vi "Launch Set Up.vi"(8 "error in (no error)":errorcluster, 11 "name or relative path":string) -> (0 "error out":errorcluster, 3 "appended path":path)   [LabVIEW 2012]
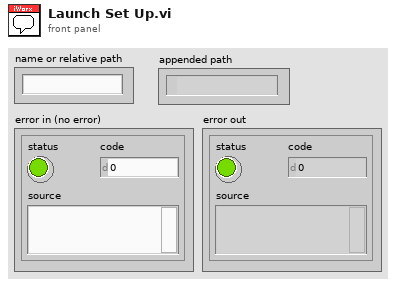
[diagram p1: front panel]
types:
  T1 = enum32{"Invalid", "Standard", "Closed", "Hidden", "Minimized", "Maximized"}
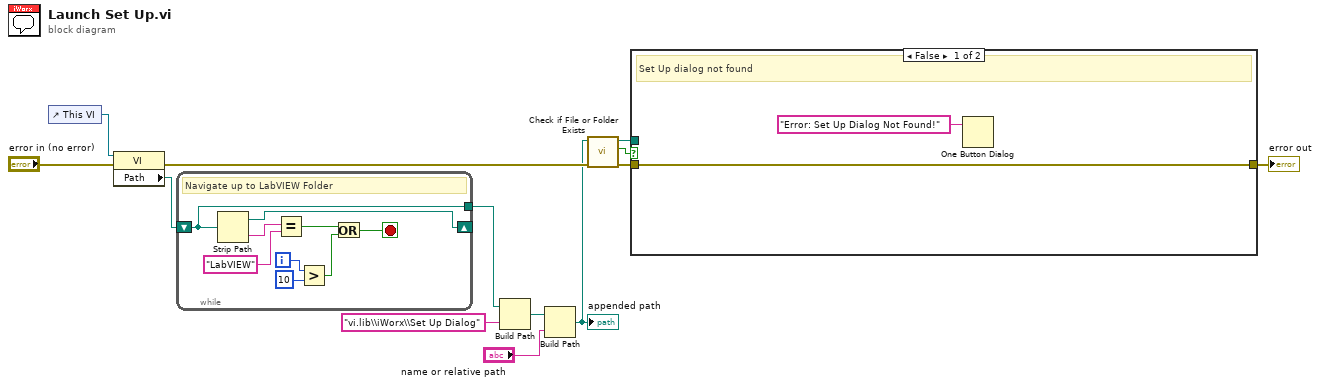
[diagram p0: block diagram]
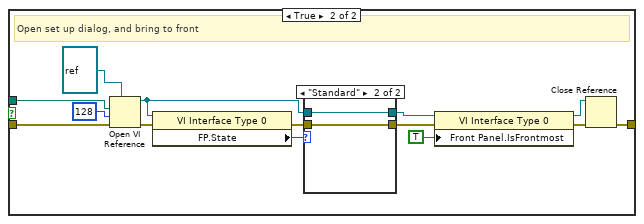
[diagram p2: hidden frame]
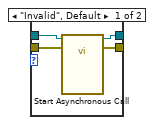
[diagram p3: hidden frame]
diagram:
  n1 = control-ref of="This VI"() -> (w8:refnum<vi>)
  n2 = property class="VI"(reference=w8, error in="error in (no error)") -> (error out=w5:errorcluster, "Path"=w9:path)  [unwired: 1 out]
  n3 = while {
    shift-right: [w22] -> _
    shift-left: w9 -> [w19]
    tunnel: [w19] -> w12
    i -> [w17]
    stop <- w14 stop-if-true
    # "Navigate up to LabVIEW Folder"
    n4 = Strip Path(path=w19) -> (stripped path=w22:path, name=w21:string)
    n5 = Equal?(x=w21, y="LabVIEW" ("name or relative path")) -> (x = y?=w18:bool)
    n6 = Greater?(x=w17, y=10) -> (0:w15:bool)
    n7 = Or(x=w18, y=w15) -> (x .or. y?=w14:bool)
  }
  n8 = Build Path(base path=w12, name or relative path="vi.lib\\iWorx\\Set Up Dialog") -> (appended path=w13:path)
  n9 = Build Path(base path=w13, name or relative path="name or relative path") -> (appended path=w4:path)
  "appended path" <- w4
  n10 = call <vilib>:"Check if File or Folder Exists.vi"("error in (no error)"=w5, "path"=w4) -> ("error out"=w2:errorcluster, "file or folder exists?"=w1:bool, "dup path"=w3:path)  [unwired: 7 in]
  n11 = case shown="False" w1 {
    tunnel: [w24 w37] -> w7
    tunnel: w3 -> [_ w35]
    tunnel: w2 -> [w24 w34]
    frame False {
      # "Set Up dialog not found"
      n12 = One Button Dialog(message="Error: Set Up Dialog Not Found!") -> ()  [unwired: 1 in, 1 out]
    }
    frame True {
      # "Open set up dialog, and bring to front"
      n13 = Open VI Reference(type specifier VI Refnum (for type only)=refnum<vi> refnum, vi path=w35, options=128, error in (no error)=w34) -> (vi reference=w28:refnum<vi>, error out=w26:errorcluster)  [unwired: 2 in]
      n14 = property class="VI Interface Type 0"(reference=w28, error in=w26) -> (error out=w25:errorcluster, "FP.State"=w27:T1)  [unwired: 1 out]
      n15 = case shown="\"Standard\"" w27 {
        tunnel: w25 -> [w42 w43]
        tunnel: [w41 w44] -> w33
        tunnel: [w40 w43] -> w31
        tunnel: w28 -> [w39 w44]
        frame "Invalid", Default {
          n16 = call-by-ref "Start Asynchronous Call"(reference=w39, error in=w42) -> (reference out=w41:refnum<vi>, error out=w40:errorcluster)  [unwired: 12 in]
        }
        frame "Standard" {
        }
      }
      n17 = property class="VI Interface Type 0"(reference=w33, error in=w31, "Front Panel.IsFrontmost"=TRUE ("Front Panel Window:Is Frontmost")) -> (reference out=w32:refnum<vi>, error out=w30:errorcluster)
      n18 = Close Reference(reference=w32, error in (no error)=w30) -> (error out=w37:errorcluster)
    }
  }
  "error out" <- w7
